vi "Drive_Initialize.vi"(11 "Drive Setup":T1={"Left Master"={"Open Data"={"SRX ID"=0, "Invert Output"=FALSE}, "Current Config Data"={"Enable Current Limit?"=FALSE, "Peak Current (Amps)"=0, "Peak Current Maximum Duration (ms)"=0, "Continuous Current Limit (Amps)"=0}, "Sensor Config"={"Feedback Device"=enum."QuadEncoder", "PhaseSensor"=FALSE}, "Hard Limits"={"Fwd Enable"=FALSE, "Rev Enable"=FALSE, "Fwd NO-NC"=enum."Normally Open", "Rev NO-NC"=enum."Normally Open"}, "Motion Magic Config Data"={"Cruise Velocity"=0, "Acceleration"=0}, "PIDF"={"P"=0.0, "I"=0.0, "D"=0.0, "F"=0.0, "I Zone"=0.0}, "Maximum Integral Accumulator Value"=0.0, "AllowableClosedLoop"=0, "Limits"={"Max"=0, "Min"=0, "Max Enable"=FALSE, "Min Enable"=FALSE}, "Output Config"={"Invert?"=FALSE, "Neutral Mode"=enum."EEPROMSetting", "Deadband (-1to1)"=0.0, "Ramp Time Off to Full (S)"=0.0, "Peak  (-1to1)"={"Forward"=1.0, "Reverse"=-1.0}, "Nominal  (-1to1)"={"Forward"=0.0, "Reverse"=0.0}}}, "Right Master"={"Open Data"={"SRX ID"=0, "Invert Output"=FALSE}, "Current Config Data"={"Enable Current Limit?"=FALSE, "Peak Current (Amps)"=0, "Peak Current Maximum Duration (ms)"=0, "Continuous Current Limit (Amps)"=0}, "Sensor Config"={"Feedback Device"=enum."QuadEncoder", "PhaseSensor"=FALSE}, "Hard Limits"={"Fwd Enable"=FALSE, "Rev Enable"=FALSE, "Fwd NO-NC"=enum."Normally Open", "Rev NO-NC"=enum."Normally Open"}, "Motion Magic Config Data"={"Cruise Velocity"=0, "Acceleration"=0}, "PIDF"={"P"=0.0, "I"=0.0, "D"=0.0, "F"=0.0, "I Zone"=0.0}, "Maximum Integral Accumulator Value"=0.0, "AllowableClosedLoop"=0, "Limits"={"Max"=0, "Min"=0, "Max Enable"=FALSE, "Min Enable"=FALSE}, "Output Config"={"Invert?"=FALSE, "Neutral Mode"=enum."EEPROMSetting", "Deadband (-1to1)"=0.0, "Ramp Time Off to Full (S)"=0.0, "Peak  (-1to1)"={"Forward"=1.0, "Reverse"=-1.0}, "Nominal  (-1to1)"={"Forward"=0.0, "Reverse"=0.0}}}, "Left Slave"={"Open Data"={"SRX ID"=0, "Invert Output"=FALSE}, "Current Config Data"={"Enable Current Limit?"=FALSE, "Peak Current (Amps)"=0, "Peak Current Maximum Duration (ms)"=0, "Continuous Current Limit (Amps)"=0}, "Sensor Config"={"Feedback Device"=enum."QuadEncoder", "PhaseSensor"=FALSE}, "Hard Limits"={"Fwd Enable"=FALSE, "Rev Enable"=FALSE, "Fwd NO-NC"=enum."Normally Open", "Rev NO-NC"=enum."Normally Open"}, "Motion Magic Config Data"={"Cruise Velocity"=0, "Acceleration"=0}, "PIDF"={"P"=0.0, "I"=0.0, "D"=0.0, "F"=0.0, "I Zone"=0.0}, "Maximum Integral Accumulator Value"=0.0, "AllowableClosedLoop"=0, "Limits"={"Max"=0, "Min"=0, "Max Enable"=FALSE, "Min Enable"=FALSE}, "Output Config"={"Invert?"=FALSE, "Neutral Mode"=enum."EEPROMSetting", "Deadband (-1to1)"=0.0, "Ramp Time Off to Full (S)"=0.0, "Peak  (-1to1)"={"Forward"=1.0, "Reverse"=-1.0}, "Nominal  (-1to1)"={"Forward"=0.0, "Reverse"=0.0}}}, "Right Slave"={"Open Data"={"SRX ID"=0, "Invert Output"=FALSE}, "Current Config Data"={"Enable Current Limit?"=FALSE, "Peak Current (Amps)"=0, "Peak Current Maximum Duration (ms)"=0, "Continuous Current Limit (Amps)"=0}, "Sensor Config"={"Feedback Device"=enum."QuadEncoder", "PhaseSensor"=FALSE}, "Hard Limits"={"Fwd Enable"=FALSE, "Rev Enable"=FALSE, "Fwd NO-NC"=enum."Normally Open", "Rev NO-NC"=enum."Normally Open"}, "Motion Magic Config Data"={"Cruise Velocity"=0, "Acceleration"=0}, "PIDF"={"P"=0.0, "I"=0.0, "D"=0.0, "F"=0.0, "I Zone"=0.0}, "Maximum Integral Accumulator Value"=0.0, "AllowableClosedLoop"=0, "Limits"={"Max"=0, "Min"=0, "Max Enable"=FALSE, "Min Enable"=FALSE}, "Output Config"={"Invert?"=FALSE, "Neutral Mode"=enum."EEPROMSetting", "Deadband (-1to1)"=0.0, "Ramp Time Off to Full (S)"=0.0, "Peak  (-1to1)"={"Forward"=1.0, "Reverse"=-1.0}, "Nominal  (-1to1)"={"Forward"=0.0, "Reverse"=0.0}}}, "Left Slave Top"={"Open Data"={"SRX ID"=0, "Invert Output"=FALSE}, "Current Config Data"={"Enable Current Limit?"=FALSE, "Peak Current (Amps)"=0, "Peak Current Maximum Duration (ms)"=0, "Continuous Current Limit (Amps)"=0}, "Sensor Config"={"Feedback Device"=enum."QuadEncoder", "PhaseSensor"=FALSE}, "Hard Limits"={"Fwd Enable"=FALSE, "Rev Enable"=FALSE, "Fwd NO-NC"=enum."Normally Open", "Rev NO-NC"=enum."Normally Open"}, "Motion Magic Config Data"={"Cruise Velocity"=0, "Acceleration"=0}, "PIDF"={"P"=0.0, "I"=0.0, "D"=0.0, "F"=0.0, "I Zone"=0.0}, "Maximum Integral Accumulator Value"=0.0, "AllowableClosedLoop"=0, "Limits"={"Max"=0, "Min"=0, "Max Enable"=FALSE, "Min Enable"=FALSE}, "Output Config"={"Invert?"=FALSE, "Neutral Mode"=enum."EEPROMSetting", "Deadband (-1to1)"=0.0, "Ramp Time Off to Full (S)"=0.0, "Peak  (-1to1)"={"Forward"=1.0, "Reverse"=-1.0}, "Nominal  (-1to1)"={"Forward"=0.0, "Reverse"=0.0}}}, "Right Slave Top"={"Open Data"={"SRX ID"=0, "Invert Output"=FALSE}, "Current Config Data"={"Enable Current Limit?"=FALSE, "Peak Current (Amps)"=0, "Peak Current Maximum Duration (ms)"=0, "Continuous Current Limit (Amps)"=0}, "Sensor Config"={"Feedback Device"=enum."QuadEncoder", "PhaseSensor"=FALSE}, "Hard Limits"={"Fwd Enable"=FALSE, "Rev Enable"=FALSE, "Fwd NO-NC"=enum."Normally Open", "Rev NO-NC"=enum."Normally Open"}, "Motion Magic Config Data"={"Cruise Velocity"=0, "Acceleration"=0}, "PIDF"={"P"=0.0, "I"=0.0, "D"=0.0, "F"=0.0, "I Zone"=0.0}, "Maximum Integral Accumulator Value"=0.0, "AllowableClosedLoop"=0, "Limits"={"Max"=0, "Min"=0, "Max Enable"=FALSE, "Min Enable"=FALSE}, "Output Config"={"Invert?"=FALSE, "Neutral Mode"=enum."EEPROMSetting", "Deadband (-1to1)"=0.0, "Ramp Time Off to Full (S)"=0.0, "Peak  (-1to1)"={"Forward"=1.0, "Reverse"=-1.0}, "Nominal  (-1to1)"={"Forward"=0.0, "Reverse"=0.0}}}}) -> (3 "RobotDriveDevRef Out":T15)   [LabVIEW 2017, in "WCDrive2018.lvlib"]
uses:
  WCDrive2018.lvlib
  <vilib>/Rock Robotics/WPI/RobotDrive/WPI_RobotDriveDevRef.ctl
  <vilib>/Rock Robotics/WPI/MotorControl/WPI_MotorControlDeviceRef.ctl
  <vilib>/Rock Robotics/WPI/MotorControl/WPI_MotorControlType.ctl
  <vilib>/Rock Robotics/SystemInterfaces/DIO/FPGA_DIOPWMChannel.ctl
  <vilib>/Rock Robotics/WPI/PWM/WPI_PWMDeadband.ctl
  <vilib>/Rock Robotics/SystemInterfaces/DIO/FPGA_DIOChannel.ctl
  TypeDef/CLUSTER_Drive_Setup.ctl
  TypeDef/CLUSTER_Talon_Setup.ctl
  _SHARE ALL/RoboRio Share All/SRX Share All/TypeDefs SRX/Cluster_SRX_OPEN Data.ctl
  _SHARE ALL/RoboRio Share All/SRX Share All/TypeDefs SRX/Cluster_SRX_Current Config.ctl
  _SHARE ALL/RoboRio Share All/SRX Share All/TypeDefs SRX/Cluster_SRX_Sensor Config.ctl
  System Drivers/Phoenix-LabVIEW/Motor Controller/Controls/CTRE_Phoenix_MotorControl_FeedbackDevice.ctl
  _SHARE ALL/RoboRio Share All/SRX Share All/TypeDefs SRX/Cluster_SRX_Config Hard Limits.ctl
  System Drivers/Phoenix-LabVIEW/Motor Controller/Controls/CTRE_Phoenix_MotorControl_LimitSwitchNormal.ctl
  _SHARE ALL/RoboRio Share All/SRX Share All/TypeDefs SRX/Cluster_SRX_Motion Magic Config Data.ctl
  _SHARE ALL/RoboRio Share All/SRX Share All/TypeDefs SRX/Cluster_SRX_PIDF.ctl
  _SHARE ALL/RoboRio Share All/SRX Share All/TypeDefs SRX/Cluster_SRX_Config Soft Limits.ctl
  _SHARE ALL/RoboRio Share All/SRX Share All/TypeDefs SRX/Cluster_SRX_Config Voltage Output.ctl
  System Drivers/Phoenix-LabVIEW/Motor Controller/Controls/CTRE_Phoenix_MotorControl_NeutralMode.ctl
  _SHARE ALL/RoboRio Share All/SRX Share All/TypeDefs SRX/Cluster_SRX_Forward and Reverse.ctl
  <vilib>/Rock Robotics/WPI/RobotDrive/WPI_RobotDriveOpen4MotorWithExistingMotors.vi
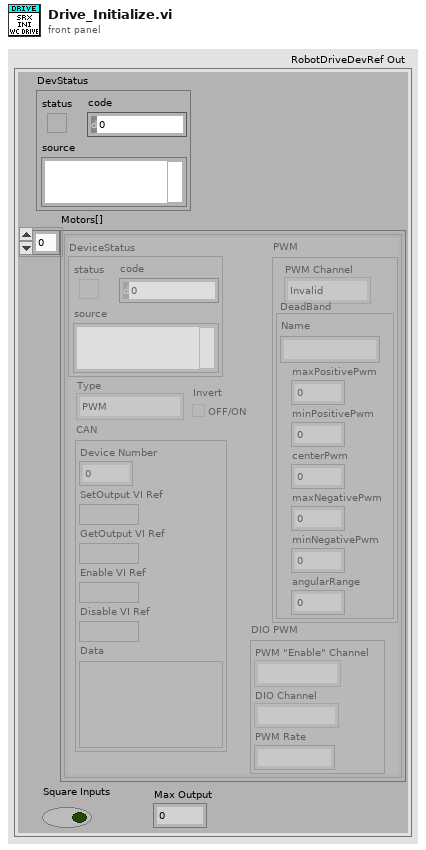
[diagram p1: front panel]
types:
  T1 = typedef "CLUSTER_Drive_Setup.ctl" = cluster{"Left Master":T2, "Right Master":T2, "Left Slave":T2, "Right Slave":T2, "Left Slave Top":T2, "Right Slave Top":T2}
  T2 = typedef "CLUSTER_Talon_Setup.ctl" = cluster{"Open Data":T3, "Current Config Data":T4, "Sensor Config":T5, "Hard Limits":T7, "Motion Magic Config Data":T9, "PIDF":T10, "Maximum Integral Accumulator Value":dbl, "AllowableClosedLoop":i32, "Limits":T11, "Output Config":T12}
  T3 = typedef "Cluster_SRX_OPEN Data.ctl" = cluster{"SRX ID":u8, "Invert Output":bool}
  T4 = typedef "Cluster_SRX_Current Config.ctl" = cluster{"Enable Current Limit?":bool, "Peak Current (Amps)":i32, "Peak Current Maximum Duration (ms)":i32, "Continuous Current Limit (Amps)":i32}
  T5 = typedef "Cluster_SRX_Sensor Config.ctl" = cluster{"Feedback Device":T6, "PhaseSensor":bool}
  T6 = typedef "CTRE_Phoenix_MotorControl_FeedbackDevice.ctl" = enum16{"None", "QuadEncoder", "Analog", "Tachometer", "Pulse Width Encoded Position", "Sensor Sum (S0 + S1)", "Sensor Difference (D0 - D1)", "Remote Source 0", "Remote Source 1", "Software Emulated"}
  T7 = typedef "Cluster_SRX_Config Hard Limits.ctl" = cluster{"Fwd Enable":bool, "Rev Enable":bool, "Fwd NO-NC":T8, "Rev NO-NC":T8}
  T8 = typedef "CTRE_Phoenix_MotorControl_LimitSwitchNormal.ctl" = enum16{"Normally Open", "Normally Closed", "Disabled"}
  T9 = typedef "Cluster_SRX_Motion Magic Config Data.ctl" = cluster{"Cruise Velocity":i32, "Acceleration":i32}
  T10 = typedef "Cluster_SRX_PIDF.ctl" = cluster{"P":dbl, "I":dbl, "D":dbl, "F":dbl, "I Zone":dbl}
  T11 = typedef "Cluster_SRX_Config Soft Limits.ctl" = cluster{"Max":i32, "Min":i32, "Max Enable":bool, "Min Enable":bool}
  T12 = typedef "Cluster_SRX_Config Voltage Output.ctl" = cluster{"Invert?":bool, "Neutral Mode":T13, "Deadband (-1to1)":dbl, "Ramp Time Off to Full (S)":dbl, "Peak  (-1to1)":T14, "Nominal  (-1to1)":T14}
  T13 = typedef "CTRE_Phoenix_MotorControl_NeutralMode.ctl" = enum8{"EEPROMSetting", "Override to Coast", "Override to Brake"}
  T14 = typedef "Cluster_SRX_Forward and Reverse.ctl" = cluster{"Forward":dbl, "Reverse":dbl}
  T15 = typedef "WPI_RobotDriveDevRef.ctl" = cluster{"DevStatus":errorcluster, "Motors[]":T16[], "Square Inputs":bool, "Max Output":dbl}
  T16 = typedef "WPI_MotorControlDeviceRef.ctl" = cluster{"DeviceStatus":errorcluster, "Type":T17, "PWM":cluster{"PWM Channel":T18, "DeadBand":T19}, "CAN":cluster{"Device Number":u8, "SetOutput VI Ref":variant, "GetOutput VI Ref":variant, "Enable VI Ref":variant, "Disable VI Ref":variant, "Data":variant}, "Invert":bool, "DIO PWM":cluster{"PWM \"Enable\" Channel":T18, "DIOChannel":T20, "PWM Rate":dbl}}
  T17 = typedef "WPI_MotorControlType.ctl" = enum16{"PWM", "CAN", "DIO PWM"}
  T18 = typedef "FPGA_DIOPWMChannel.ctl" = enum8{"PWM 0", "PWM 1", "PWM 2", "PWM 3", "PWM 4", "PWM 5", "PWM 6", "PWM 7", "PWM 8", "PWM 9", "PWM MXP 0", "PWM MXP 1", "PWM MXP 2", "PWM MXP 3", "PWM MXP 4", "PWM MXP 5", "PWM MXP 6", "PWM MXP 7", "PWM MXP 8", "PWM MXP 9", "Invalid"}
  T19 = typedef "WPI_PWMDeadband.ctl" = cluster{"Name":string, "maxPositivePwm":i32, "minPositivePwm":i32, "centerPwm":i32, "maxNegativePwm":i32, "minNegativePwm":i32, "angularRange":u16}
  T20 = typedef "FPGA_DIOChannel.ctl" = enum8{"DIO 0", "DIO 1", "DIO 2", "DIO 3", "DIO 4", "DIO 5", "DIO 6", "DIO 7", "DIO 8", "DIO 9", "DIO MXP 0", "DIO MXP 1", "DIO MXP 2", "DIO MXP 3", "DIO MXP 4", "DIO MXP 5", "DIO MXP 6", "DIO MXP 7", "DIO MXP 8", "DIO MXP 9", "DIO MXP 10", "DIO MXP 11", "DIO MXP 12", "DIO MXP 13", "DIO MXP 14", "DIO MXP 15", "SPI Port CS1", "SPI Port CS2", "SPI Port CS3", "SPI Port MISO", "SPI Port MOSI", "Invalid"}
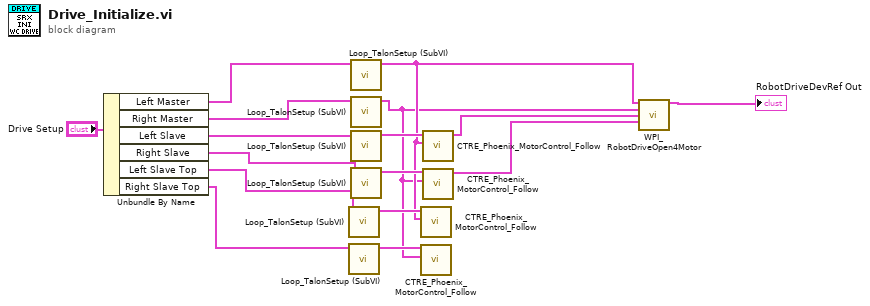
[diagram p0: block diagram]
diagram:
  n1 = Unbundle By Name("Drive Setup") -> ("Left Master"=w14:T2, "Right Master"=w13:T2, "Left Slave"=w12:T2, "Right Slave"=w11:T2, "Left Slave Top"=w2:T2, "Right Slave Top"=w1:T2)
  n2 = call "Loop_TalonSetup (SubVI).vi"("Talon Setup"=w2) -> ("PhoenixMotorControlDevRef"=w5:T16)  [unwired: 10 in]
  n3 = call "Loop_TalonSetup (SubVI).vi"("Talon Setup"=w1) -> ("PhoenixMotorControlDevRef"=w6:T16)  [unwired: 10 in]
  n4 = call "Loop_TalonSetup (SubVI).vi"("Talon Setup"=w14) -> ("PhoenixMotorControlDevRef"=w4:T16)  [unwired: 10 in]
  n5 = call "Loop_TalonSetup (SubVI).vi"("Talon Setup"=w13) -> ("PhoenixMotorControlDevRef"=w3:T16)  [unwired: 10 in]
  n6 = call "Loop_TalonSetup (SubVI).vi"("Talon Setup"=w12) -> ("PhoenixMotorControlDevRef"=w9:T16)  [unwired: 10 in]
  n7 = call "Loop_TalonSetup (SubVI).vi"("Talon Setup"=w11) -> ("PhoenixMotorControlDevRef"=w10:T16)  [unwired: 10 in]
  n8 = call "CTRE_Phoenix_MotorControl_Follow.vi"("Master Controller to Follow"=w4, "PhoenixMotorControlDevRef"=w5) -> ()  [unwired: 8 in, 2 out]
  n9 = call "CTRE_Phoenix_MotorControl_Follow.vi"("Master Controller to Follow"=w3, "PhoenixMotorControlDevRef"=w6) -> ()  [unwired: 8 in, 2 out]
  n10 = call "CTRE_Phoenix_MotorControl_Follow.vi"("Master Controller to Follow"=w4, "PhoenixMotorControlDevRef"=w9) -> ("PhoenixMotorControlDevRef"=w8:T16)  [unwired: 8 in, 1 out]
  n11 = call "CTRE_Phoenix_MotorControl_Follow.vi"("Master Controller to Follow"=w3, "PhoenixMotorControlDevRef"=w10) -> ("PhoenixMotorControlDevRef"=w7:T16)  [unwired: 8 in, 1 out]
  n12 = call-poly <vilib>:"WPI_RobotDriveOpen4Motor.vi"("Rear Left Motor Dev Ref"=w4, "Rear Right Motor Dev Ref"=w3, "Front Left Motor Dev Ref"=w8, "Front Right Motor Dev Ref"=w7) -> ("RobotDriveDevRef"=→"RobotDriveDevRef Out":T15)  [unwired: 10 in, 1 out]
